vi "Max Robot Speed.vi"() -> ()   [LabVIEW 2012]
panel:
  in  "Max Speed":dbl=29000.0
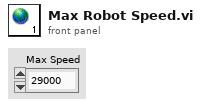
[diagram p1: front panel]
diagram:
